vi "ex_UI_SupportTDMS.vi"() -> (1 "support TDMSû":bool=TRUE)   [LabVIEW 2017]
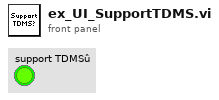
[diagram p1: front panel]
types:
  T1 = enum32{"invalid OS target", "Mac OS", "Windows 3.1", "Windows 95/NT", "Solaris 1", "Solaris 2", "HP-UX", "PowerMAX", "Linux", "Irix", "Rhapsody", "BeOS", "AIX", "OSF1", "VxWorks", "PharLap", "Carbon", "RTX", "Windows x64", "Linux x64", "Mac OS X x64"}
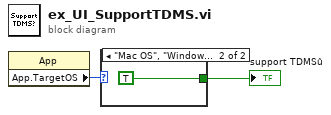
[diagram p0: block diagram]
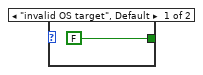
[diagram p2: hidden frame]
diagram:
  n1 = property class="App"() -> ("App.TargetOS"=w2:T1)  [unwired: 2 in, 2 out]
  n2 = case shown="\"Mac OS\", \"Windows 95/NT\", \"Linux\", \"Carbon\", \"Windows x64\"..\"Mac OS X x64\"" w2 {
    tunnel: [FALSE TRUE] -> w1
    frame "invalid OS target", Default {
    }
    frame "Mac OS", "Windows 95/NT", "Linux", "Carbon", "Windows x64".."Mac OS X x64" {
    }
  }
  "support TDMSû" <- w1
